vi "LinxUartWrite.vi"(8 "Error In":errorcluster, 9 "Data":u8[](array[numeric]), 10 "Uart Channel":u8, 11 "LINX Resource":T1) -> (0 "Error Out":errorcluster, 3 "LINX Resource":T1)   [LabVIEW 2014, in "LMH-LINX.lvlib" / "Local IO.lvlib"]
uses:
  <vilib>/MakerHub/LINX/Private/Local IO/Local IO.lvlib
  <vilib>/MakerHub/LINX/Private/Type Defs/LINX Ref.ctl
  <vilib>/MakerHub/LINX/Private/Type Defs/Platform.ctl
  <vilib>/MakerHub/LINX/Private/Type Defs/Interface.ctl
  <vilib>/MakerHub/LINX/Private/Device/Type Defs/LINX Device Config.ctl
  <vilib>/MakerHub/LINX/Private/Device/Type Defs/TCP Config.ctl
  <vilib>/MakerHub/LINX/Private/Device/Type Defs/Channels.ctl
  <vilib>/MakerHub/LINX/Private/Type Defs/Error Type.ctl
  <vilib>/MakerHub/LINX/LMH-LINX.lvlib
  <vilib>/MakerHub/LINX/Private/Type Defs/Channel FGV States.ctl
  liblinxdevice.dll
  <vilib>/MakerHub/LINX/Private/Device/Device.lvlib
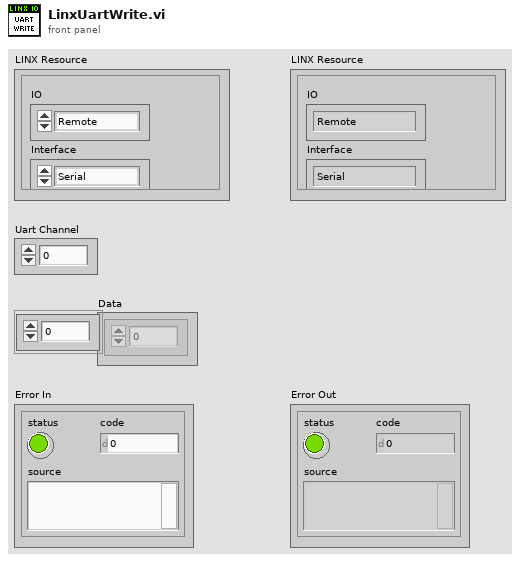
[diagram p1: front panel]
types:
  T1 = typedef "LMH-LINX.lvlib/LINX Ref.ctl" = cluster{"IO":T2, "Interface":T3, "LINX Device Config":T4}
  T2 = typedef "LMH-LINX.lvlib/Platform.ctl" = enum16{"Remote", "Local"}
  T3 = typedef "LMH-LINX.lvlib/Interface.ctl" = enum16{"Serial", "TCP"}
  T4 = typedef "LMH-LINX.lvlib/Device.lvlib/LINX Device Config.ctl" = cluster{"Interface":T3, "COM Port":refnum<visa-resource-name>, "TCP Configuration":T5, "Device Family":u8, "Device ID":u8, "Device Name":string, "TCP Ref":refnum<k5>, "Channels":T6}
  T5 = typedef "LMH-LINX.lvlib/Device.lvlib/TCP Config.ctl" = cluster{"IP Address":string, "Port":u16}
  T6 = typedef "LMH-LINX.lvlib/Channels.ctl" = cluster{"DI":u8[], "DO":u8[], "AI":u8[], "AO":u8[], "PWM":u8[], "QE":u8[], "UART":u8[], "I2C 2":u8[], "SPI":u8[], "CAN":u8[], "Servo":u8[], "AI Ref (V)":dbl, "AI Resolution (Bits)":u8, "AO Ref (V)":dbl, "AO Resolution (Bits)":u8}
  T7 = typedef "LMH-LINX.lvlib/Error Type.ctl" = enum16{"Unknown", "Timeout", "Corrupt Return Packet", "Unable To Connect", "Command Not Supported", "Channel DNE", "Invalid COM Config", "Firmware Version Mismatch", "myRIO Support", "CMD Specific Error", "Local IO Not Supported"}
  T8 = typedef "LMH-LINX.lvlib/Channel FGV States.ctl" = enum16{"Initialize", "Get", "Set"}
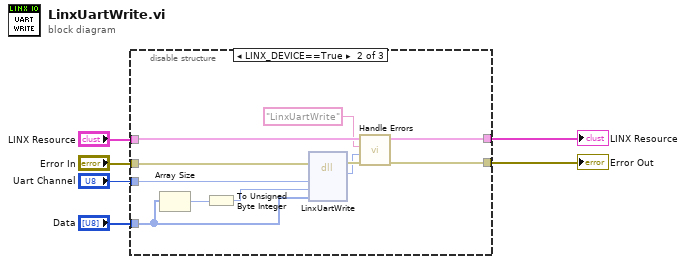
[diagram p0: block diagram]
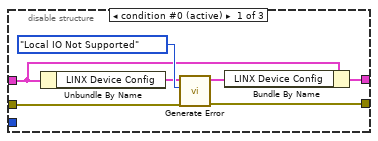
[diagram p2: hidden frame]
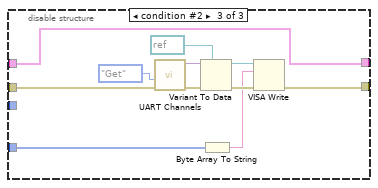
[diagram p3: hidden frame]
diagram:
  n1 = disable-structure shown="LINX_DEVICE==True" {
    disable-tunnel: [w7 w21 w35] -> w5
    disable-tunnel: "LINX Resource" -> [w9 w22 w35]
    disable-tunnel: "Error In" -> [w12 w24 w27]
    disable-tunnel: [w11 w19 w26] -> w6
    disable-tunnel: "Uart Channel" -> [_ w23 _]
    disable-tunnel: "Data" -> [_ w16 w25]
    frame condition #0 (active) {
      n2 = Unbundle By Name(w9) -> ("LINX Device Config"=w10:T4)
      n3 = call <vilib>:"Generate Error.vi"("Error In"=w12, "Error Type"=Error_Type."Local IO Not Supported", "LINX Device Config"=w10) -> ("Error Out"=w11:errorcluster, "Dup LINX Device Config"=w8:T4)  [unwired: 7 in]
      n4 = Bundle By Name(cluster=w9, "LINX Device Config"=w8) -> (w7:T1)
    }
    frame condition #1 {
      n5 = Array Size(array=w16) -> (size(s)=w15:i32)
      n6 = To Unsigned Byte Integer(number=w15) -> (unsigned 8bit integer=w14:u8)
      n7 = dll-call lib="liblinxdevice.*" fn="LinxUartWrite"(error in=w24, "channel"=w23, "numBytes"=w14, "sendBuffer"=w16) -> (error out=w20:errorcluster, "status"=w17:i32)  [unwired: 5 in, 1 out]
      n8 = call <vilib>:"Handle Errors.vi"("Error In"=w20, "LinxStatus"=w17, "Function Name"="LinxUartWrite", "LINX Resource"=w22) -> ("Error Out"=w19:errorcluster, "LINX Resource"=w21:T1)  [unwired: 6 in]
    }
    frame condition #2 {
      n9 = call <vilib>:"UART Channels.vi"("Error In"=w27, "Channel State"=Channel_FGV_States."Get") -> ("Error Out"=w34:errorcluster, "UART Channel"=w33:variant)  [unwired: 8 in]
      n10 = Variant To Data(error in=w34, type=refnum<visa-resource-name> refnum ("reference"), Variant=w33) -> (data=w29:refnum<visa-resource-name>, error out=w30:errorcluster)
      n11 = Byte Array To String(unsigned byte array=w25) -> (string=w28:string)
      n12 = VISA Write(VISA resource name=w29, write buffer=w28, error in (no error)=w30) -> (error out=w26:errorcluster)  [unwired: 2 out]
    }
  }
  "LINX Resource" <- w5
  "Error Out" <- w6
